vi "Scan Serial Number.vi"() -> (1 "Serial Number Out":string, 2 "OK?":bool)   [LabVIEW 2026]
panel:
  out "Original":string
  out "Prompt":string
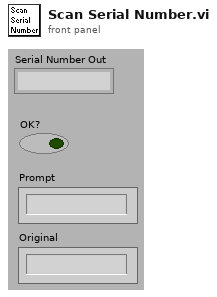
[diagram p1: front panel]
types:
  T1 = typedef "Serial Type.ctl" = enum16{"Unknown", "Tube Serial", "HE Serial", "CAP Serial"}
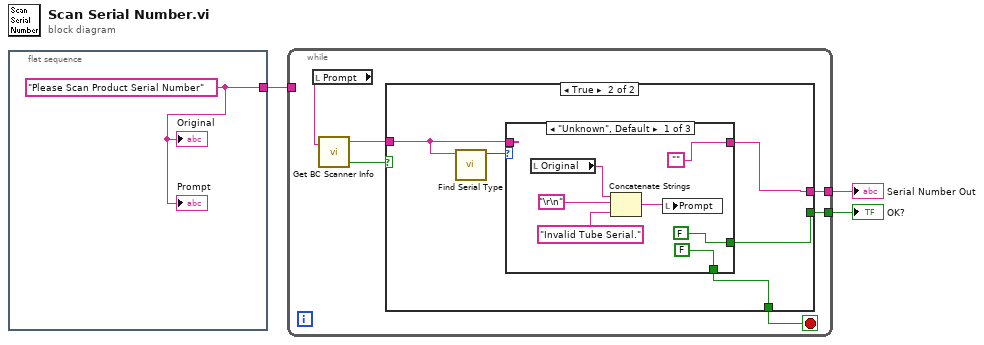
[diagram p0: block diagram]
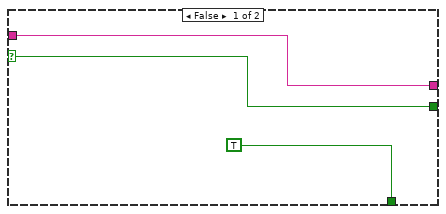
[diagram p2: hidden frame]
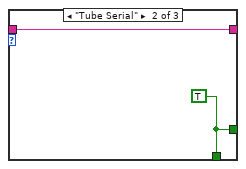
[diagram p3: hidden frame]
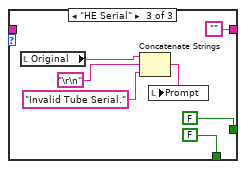
[diagram p4: hidden frame]
diagram:
  n1 = flat-sequence {
    tunnel: [w4] -> w1
    frame #0 {
      w4 = "Please Scan Product Serial Number" ("Prompt")
      "Original" <- w4
      "Prompt" <- w4
    }
  }
  n2 = while {
    tunnel: [w8] -> w2
    tunnel: [w7] -> w3
    tunnel: w1 -> [_]
    stop <- w6 stop-if-true
    n3 = local read "Prompt"() -> (w5:string)
    n4 = call "Get BC Scanner Info.vi"("Prompt"=w5) -> ("Info Out"=w9:string, "OK"=w10:bool)  [unwired: 2 in]
    n5 = case shown="True" w10 {
      selector: w10 -> [w13 _]
      tunnel: w9 -> [w12 w17]
      tunnel: [w13 w15] -> w8
      tunnel: [w12 w16] -> w7
      tunnel: [TRUE w14] -> w6
      frame False {
      }
      frame True {
        n6 = call "Find Serial Type.vi"("Serial IN"=w17) -> ("Serial Type Out"=w18:T1)  [unwired: 9 in, 1 out]
        n7 = case shown="\"Unknown\", Default" w18 {
          tunnel: w17 -> [_ w27 _]
          tunnel: ["" w27 ""] -> w16
          tunnel: [FALSE w26 FALSE] -> w15
          tunnel: [FALSE w26 FALSE] -> w14
          frame "Unknown", Default {
            n8 = local read "Original"() -> (w21:string)
            n9 = Concatenate Strings(w21, "\r\n", "Invalid Tube Serial.") -> (w19:string)
            n10 = local write "Prompt"(w19) -> ()
          }
          frame "Tube Serial" {
            w26 = TRUE
          }
          frame "HE Serial" {
            n11 = local read "Original"() -> (w30:string)
            n12 = Concatenate Strings(w30, "\r\n", "Invalid Tube Serial.") -> (w28:string)
            n13 = local write "Prompt"(w28) -> ()
          }
        }
      }
    }
  }
  "Serial Number Out" <- w3
  "OK?" <- w2
